vi "GLOBAL1.vi"() -> ()   [LabVIEW 2018]
uses:
  GLOBAL DATA INITIALIZE.vi
panel:
  in  "Boolean":bool
  in  "Knob":dbl(knob) scale=0.0..100.0
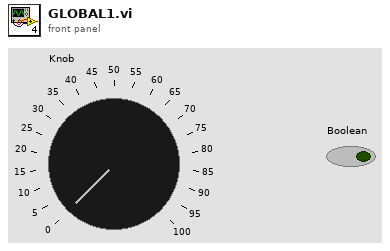
[diagram p1: front panel]
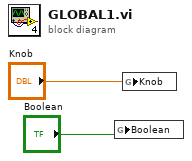
[diagram p0: block diagram]
diagram:
  n1 = global write "GLOBAL DATA INITIALIZE.vi" "Boolean"("Boolean") -> ()
  n2 = global write "GLOBAL DATA INITIALIZE.vi" "Knob"("Knob") -> ()
